vi "GlobalSetGetParametersAvantes.vi"() -> ()   [LabVIEW 2013]
panel:
  in  "SetGetParConfign":T1
  in  "AVS_Init":i32
  in  "strBuf":string
  in  "l_pPixelWavelen":dbl[](array[numeric])
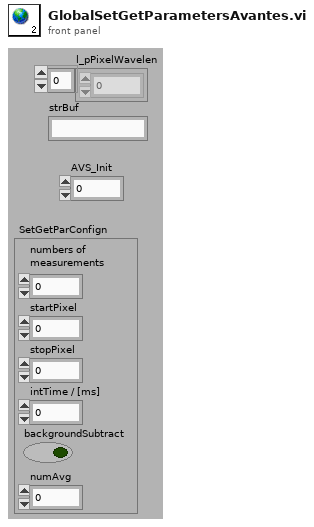
[diagram p1: front panel]
types:
  T1 = cluster{"numbers of \nmeasurements":i16, "startPixel":u16, "stopPixel":u16, "intTime / [ms]":sgl, "backgroundSubtract":bool, "numAvg":u32}
diagram:
